vi "IntToIP (SubVI).vi"(11 "Numeric":u32 format="%x") -> (3 "IP_PC":string)   [LabVIEW 2017]
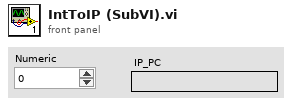
[diagram p1: front panel]
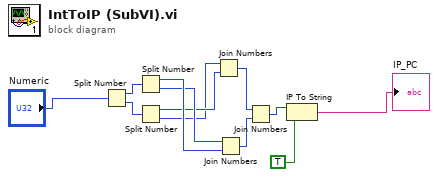
[diagram p0: block diagram]
diagram:
  n1 = Split Number(x="Numeric") -> (hi(x)=w5:u16, lo(x)=w6:u16)
  n2 = Split Number(x=w5) -> (hi(x)=w10:u8, lo(x)=w9:u8)
  n3 = Split Number(x=w6) -> (hi(x)=w8:u8, lo(x)=w7:u8)
  n4 = Join Numbers(hi=w7, lo=w8) -> ((hi.lo)=w11:u16)
  n5 = Join Numbers(hi=w9, lo=w10) -> ((hi.lo)=w12:u16)
  n6 = Join Numbers(hi=w11, lo=w12) -> ((hi.lo)=w3:u32)
  n7 = IP To String(1:TRUE ("dot notation? (F)"), 2:w3) -> (0:→"IP_PC":string)
